vi "ShooterStateMachine.vi"(0 "Shoot Button":bool, 1 "FeederSpeedDemand":dbl, 2 "ShooterSpeedDemand":dbl, 5 "ShooterSpeedThreshold":dbl, 7 "Rev Button":bool, 9 "Target Shooter Speed":dbl, 11 "BeltSpeedDemand":dbl, 12 "State":i32) -> (4 "ShooterSpeed":dbl, 6 "FeederSpeed":dbl, 8 "BeltSpeed":dbl, 15 "NextState":i32)   [LabVIEW 2020]
uses:
  AuxGlobals.vi
  <vilib>/Utility/semaphor.llb/Obtain Semaphore Reference.vi
  <vilib>/Rock Robotics/WPI/ThirdParty/JAS_Junk/TrajLib/Timer_Reset.vi
  <vilib>/Rock Robotics/WPI/ThirdParty/JAS_Junk/TrajLib/Trajectory_Library.lvlib
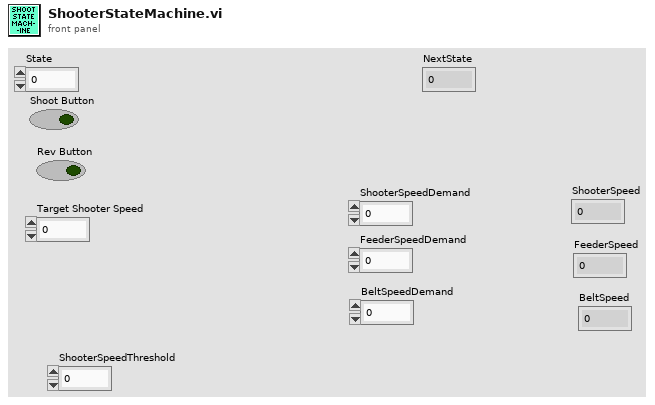
[diagram p1: front panel]
types:
  T1 = typedef "Trajectory_Library.lvlib/TIMER.ctl" = cluster{"StartTime":dbl, "Accumulated TIme":dbl, "Running":bool, "semaphore":T2}
  T2 = typedef "Semaphore RefNum" = refnum<k1>
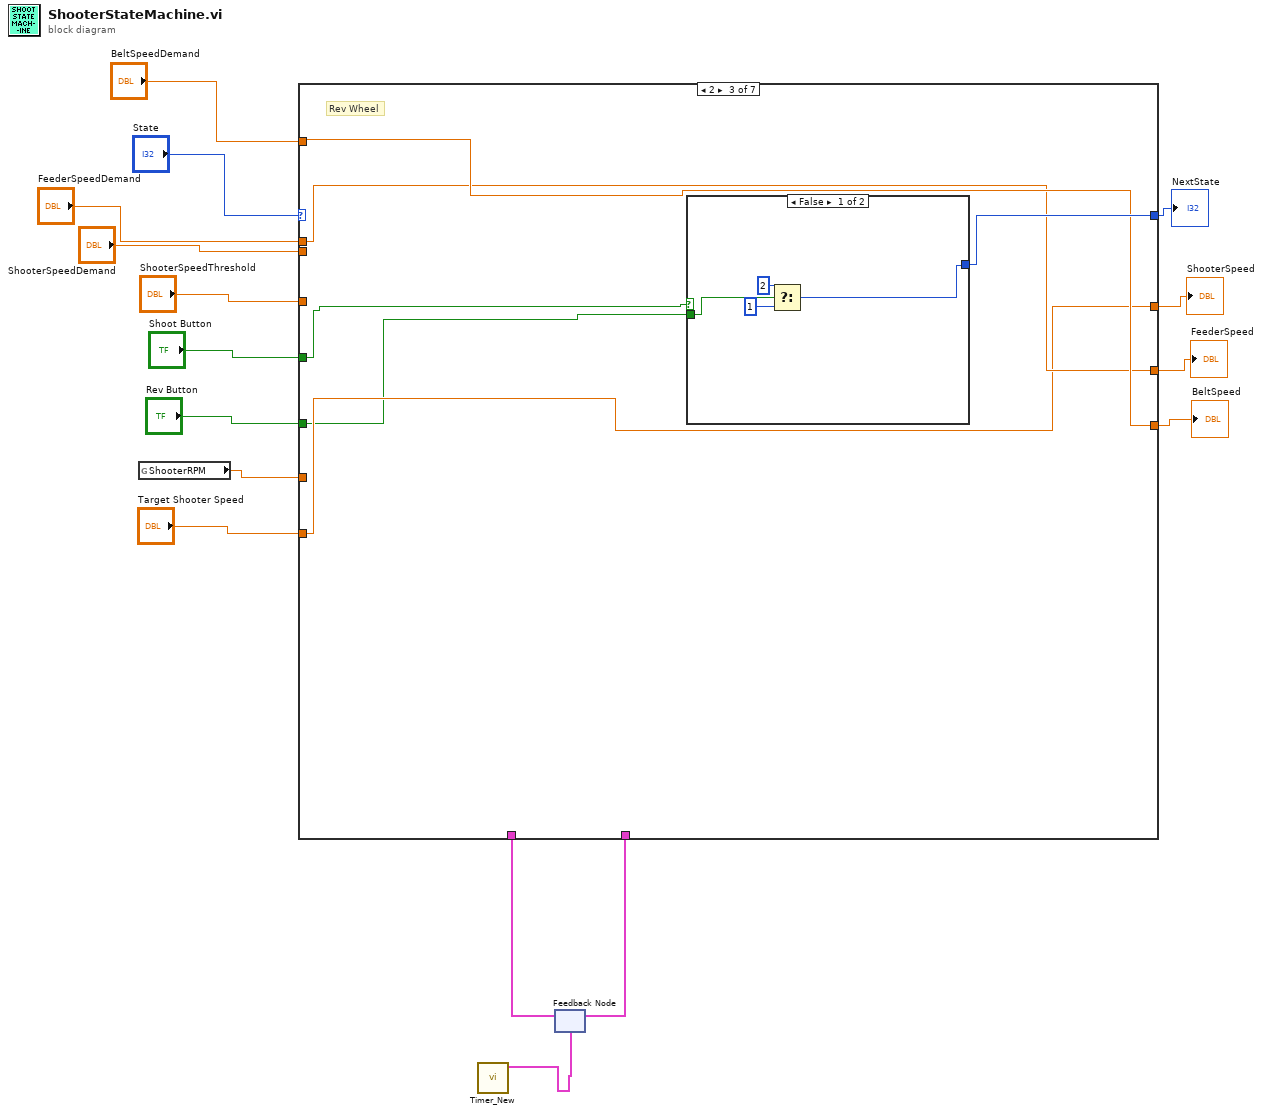
[diagram p0: block diagram]
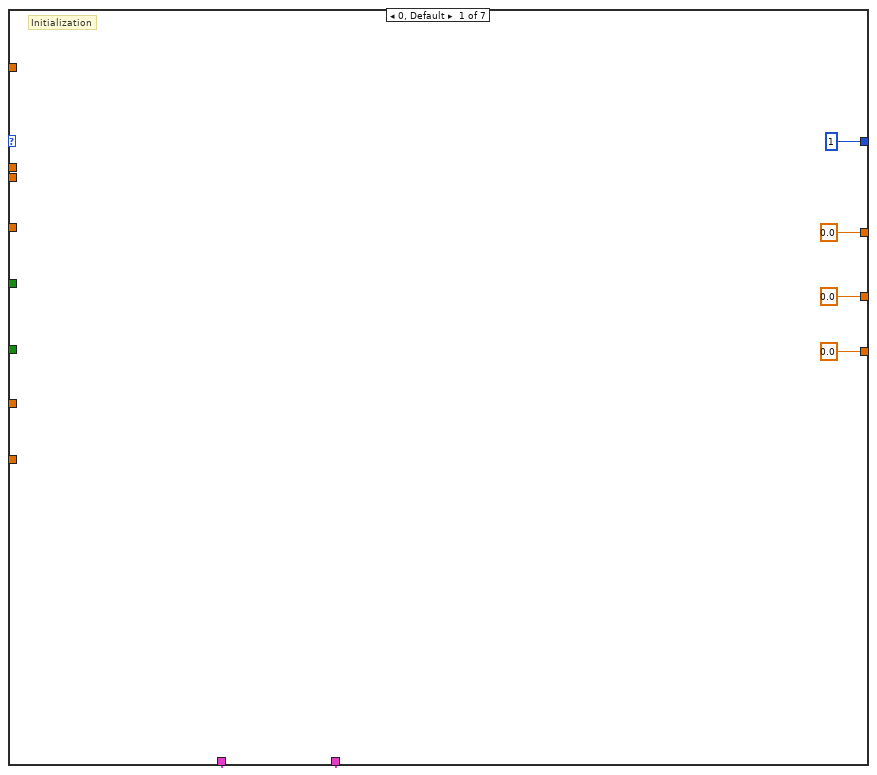
[diagram p2: hidden frame]
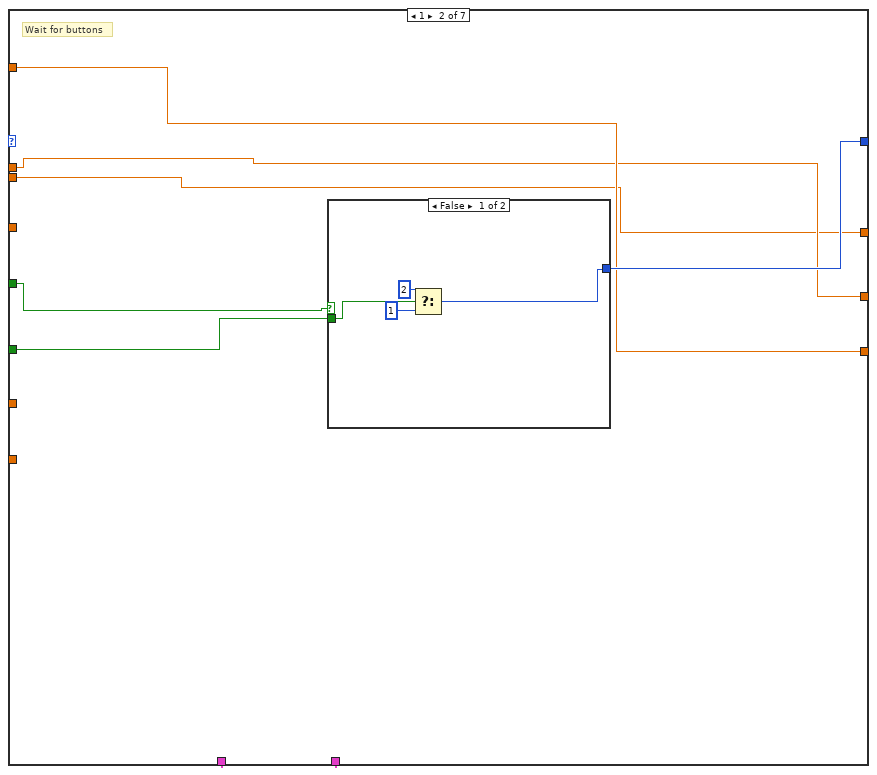
[diagram p3: hidden frame]
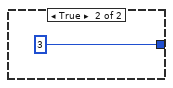
[diagram p4: hidden frame]
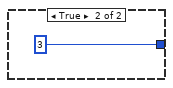
[diagram p5: hidden frame]
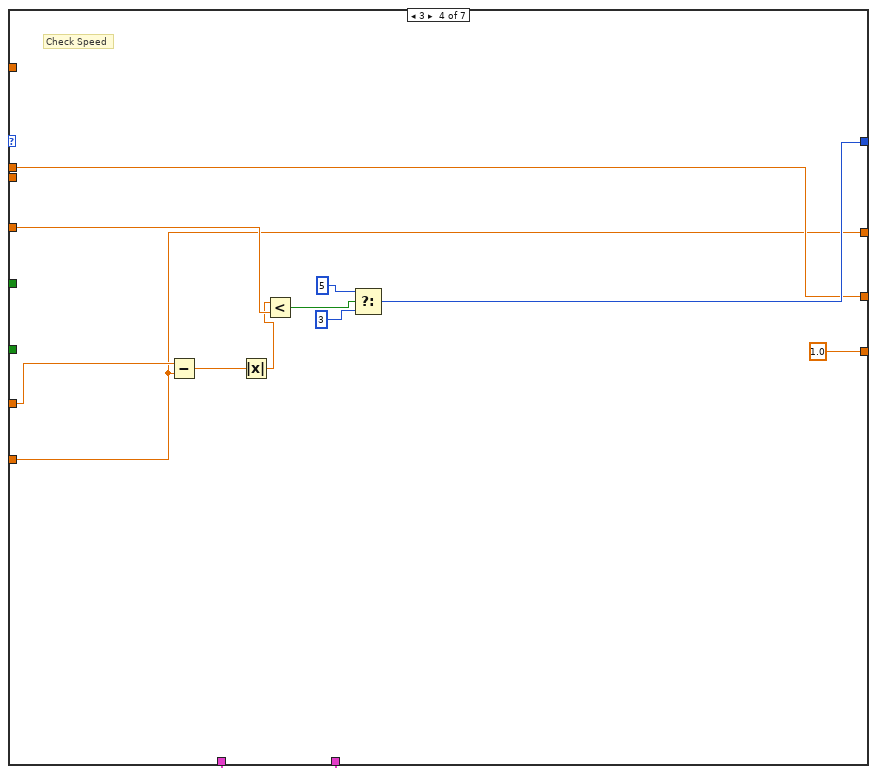
[diagram p6: hidden frame]
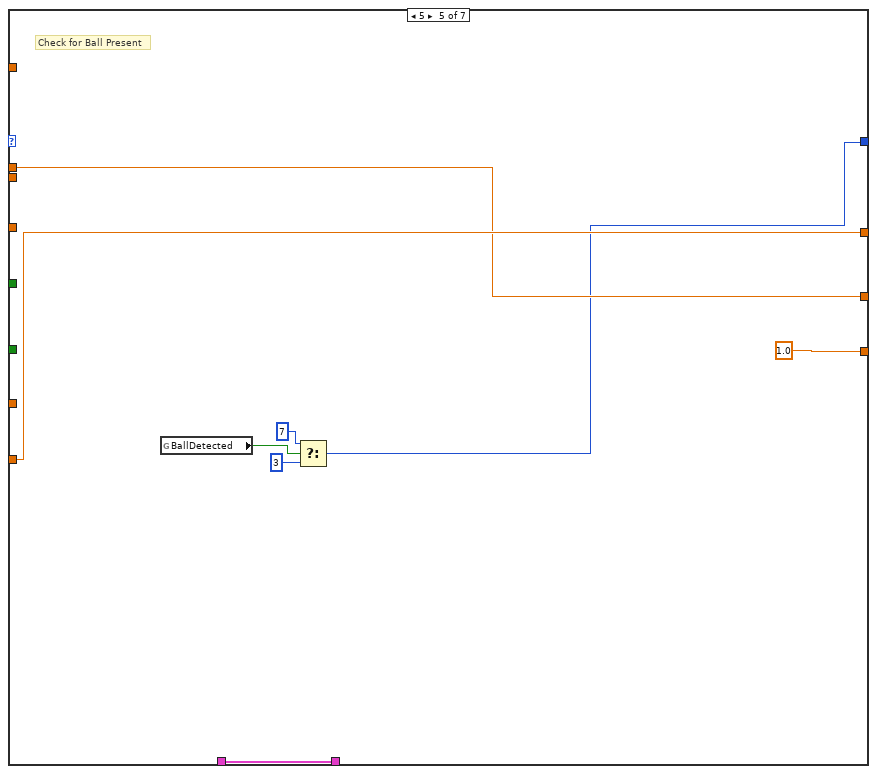
[diagram p7: hidden frame]
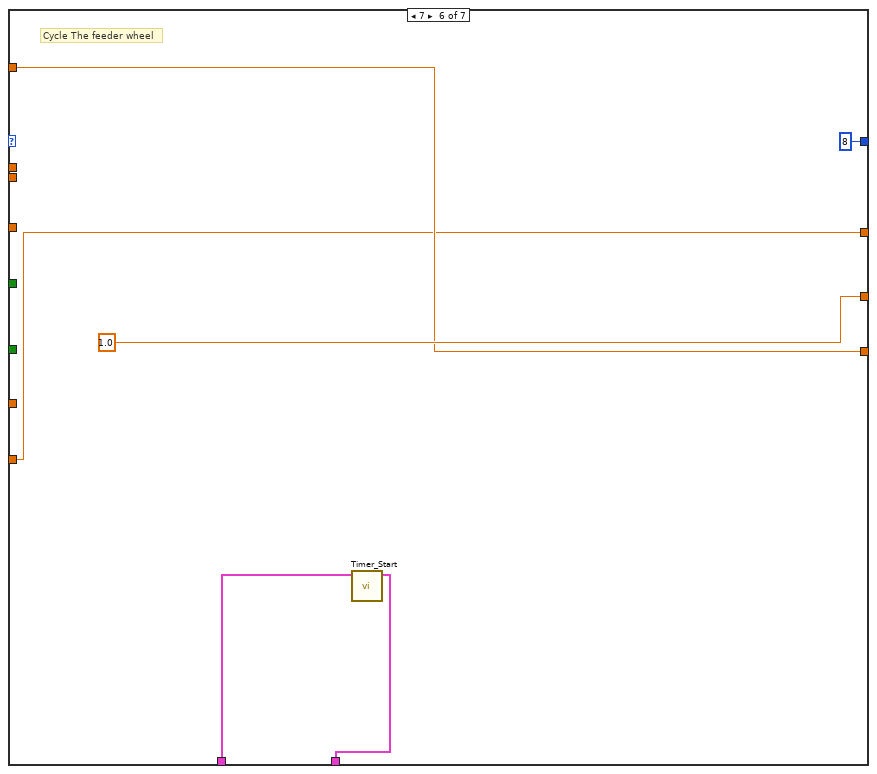
[diagram p8: hidden frame]
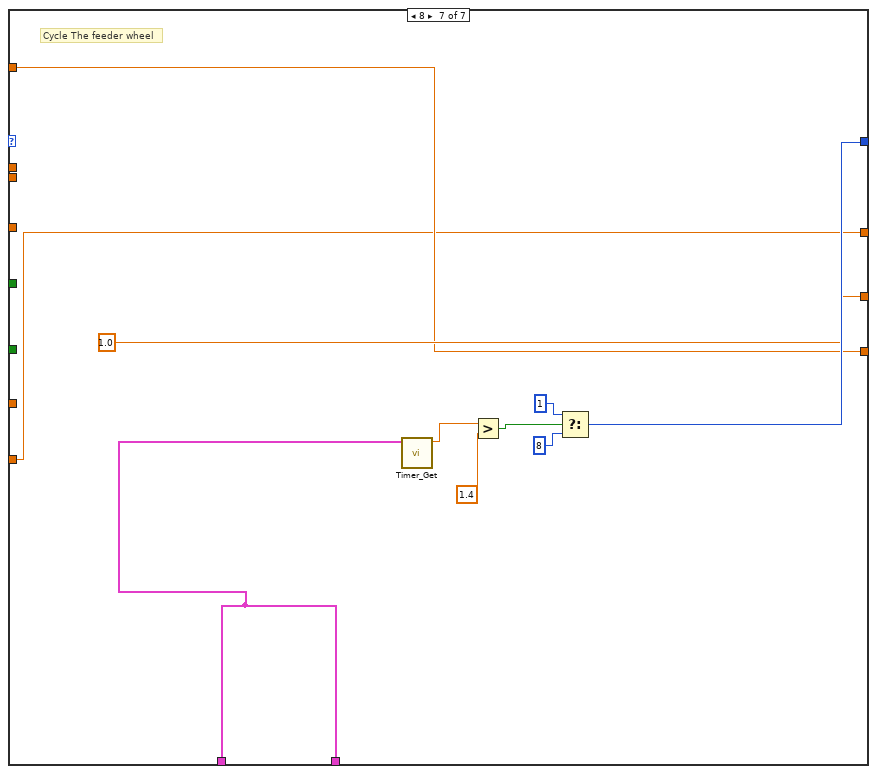
[diagram p9: hidden frame]
diagram:
  n1 = global read "AuxGlobals.vi" "ShooterRPM"() -> (w12:dbl)
  n2 = call <vilib>:"Timer_New.vi"() -> ("TIMER"=w1:T1)  [unwired: 11 in]
  n3 = feedback #1(w1) -> (w2:T1)
  n4 = case shown="2" "State" {
    tunnel: [1 w28 w40 w50 w63 8 ("f") w79] -> w15
    tunnel: "Rev Button" -> [_ w22 w35 _ _ _ _]
    tunnel: "Shoot Button" -> [_ w23 w34 _ _ _ _]
    tunnel: w12 -> [_ _ _ w57 _ _ _]
    tunnel: "Target Shooter Speed" -> [_ _ w37 w48 w65 w69 w74]
    tunnel: "ShooterSpeedThreshold" -> [_ _ _ w54 _ _ _]
    tunnel: "BeltSpeedDemand" -> [_ w27 w39 _ _ w70 w75]
    tunnel: "FeederSpeedDemand" -> [_ w26 w38 w49 w64 _ _]
    tunnel: "ShooterSpeedDemand" -> [_ w25 _ _ _ _ _]
    tunnel: [0.0 ("BeltSpeedDemand") w27 w39 1.0 ("BeltSpeedDemand") 1.0 ("BeltSpeedDemand") w70 w75] -> w6
    tunnel: [0.0 ("FeederSpeedDemand") w26 w38 w49 w64 1.0 ("FeederSpeedDemand") 1.0 ("FeederSpeedDemand")] -> w5
    tunnel: [0.0 ("ShooterSpeedDemand") w25 w37 w48 w65 w69 w74] -> w4
    tunnel: [w17 w24 w36 w47 w58 w66 w72] -> w3
    tunnel: w2 -> [w17 w24 w36 w47 w58 w67 w72]
    frame 0, Default {
      # "Initialization"
    }
    frame 1 {
      # "Wait for buttons"
      n5 = case shown="False" w23 {
        tunnel: [w29 3] -> w28
        tunnel: w22 -> [w32 _]
        frame False {
          n6 = Select(t=2, s=w32, f=1) -> (s? t:f=w29:i32)
        }
        frame True {
        }
      }
    }
    frame 2 {
      # "Rev Wheel"
      n7 = case shown="False" w34 {
        tunnel: [w41 3] -> w40
        tunnel: w35 -> [w44 _]
        frame False {
          n8 = Select(t=2, s=w44, f=1) -> (s? t:f=w41:i32)
        }
        frame True {
        }
      }
    }
    frame 3 {
      # "Check Speed"
      n9 = Subtract(x=w57, y=w48) -> (x-y=w56:dbl)
      n10 = Absolute Value(x=w56) -> (abs(x)=w53:dbl)
      n11 = Less?(x=w53, y=w54) -> (x < y?=w55:bool)
      n12 = Select(t=5, s=w55, f=3) -> (s? t:f=w50:i32)
    }
    frame 5 {
      # "Check for Ball Present"
      n13 = global read "AuxGlobals.vi" "BallDetected"() -> (w60:bool)
      n14 = Select(t=7, s=w60, f=3) -> (s? t:f=w63:i32)
    }
    frame 7 {
      # "Cycle The feeder wheel"
      n15 = call <vilib>:"Timer_Start.vi"("in Timer"=w67) -> ("out Timer"=w66:T1)  [unwired: 10 in]
    }
    frame 8 {
      # "Cycle The feeder wheel"
      n16 = call <vilib>:"Timer_Get.vi"("TIMER"=w72) -> ("CurrentTImer"=w73:dbl)  [unwired: 10 in]
      n17 = Greater?(x=w73, y=1.4) -> (0:w78:bool)
      n18 = Select(t=1, s=w78, f=8) -> (s? t:f=w79:i32)
    }
  }
  "NextState" <- w15
  "BeltSpeed" <- w6
  "FeederSpeed" <- w5
  "ShooterSpeed" <- w4
  n19 = feedback-in #1(w3) -> ()
